vi "Append VI List of SubVIs to Report (refnum).vi"(0 "report in":refnum<class "NI_report.lvclass">, 2 "image format (jpeg)":enum32{"PNG", "JPEG", "GIF"}(ring)=enum."JPEG", 5 "VI":refnum<vi>, 7 "alignment (default)":T2, 9 "include Express VI configuration information (F)":bool, 11 "error in (no error)":errorcluster, 12 "MS Office parameters":T1) -> (4 "report out":refnum<class "NI_report.lvclass">, 6 "VI out":refnum<vi>, 8 "start out (Word)":i32, 10 "end out (Word)":i32, 15 "error out":errorcluster)   [LabVIEW 2020, in "NI_ReportGenerationCore.lvlib"]
doc: "Appends a list of subVIs of the VI you specify in <B>VI</B> to a report. The list includes subVI icons, names, and paths. Wire data to the <B>VI</B> input to determine the polymorphic instance to use or manually select the instance."
uses:
  <vilib>/Utility/NIReport.llb/NI_ReportGenerationCore.lvlib
  <vilib>/Utility/NIReport.llb/NI_report.lvclass
  <vilib>/Utility/NIReport.llb/HTML Report Image Alignment.ctl
  <vilib>/printing/ReportDocExtensions.llb/File_types_for_reports.ctl
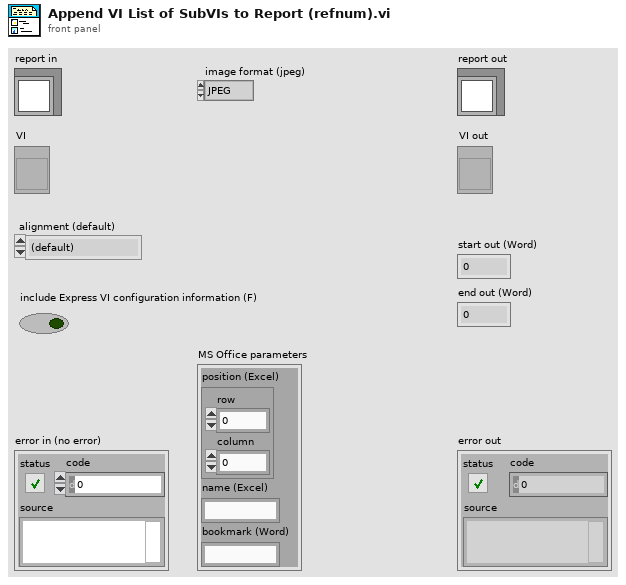
[diagram p1: front panel]
types:
  T1 = cluster{"position (Excel)":cluster{"row":i32, "column":i32}, "name (Excel)":string, "bookmark (Word)":string}
  T2 = typedef "NI_ReportGenerationCore.lvlib/HTML Report Image Alignment.ctl" = enum16{"(default)", "LEFT", "RIGHT", "TOP", "TEXTTOP", "MIDDLE", "ABSMIDDLE", "BASELINE", "BOTTOM", "ABSBOTTOM"}
  T3 = enum8{"No dynamic dispatch VIs", "Include nearest implementation", "Include all overrides"}
  T4 = typedef "NI_ReportGenerationCore.lvlib/File_types_for_reports.ctl" = enum16{".jpg", ".png", ".html", ".gif"}
  T5 = enum32{"invalid app kind", "Development System", "Run Time System", "Student Edition", "Embedded LabVIEW", "Evaluation", "Custom"}
  T6 = enum32{"invalid VI type", "Standard VI", "Control VI", "Global VI", "Polymorphic VI", "Configuration VI", "SubSystem", "Facade VI", "Method VI", "Statechart Diagram VI"}
  T7 = enum16{"Standard Report", "HTML", "Word", "Excel"}
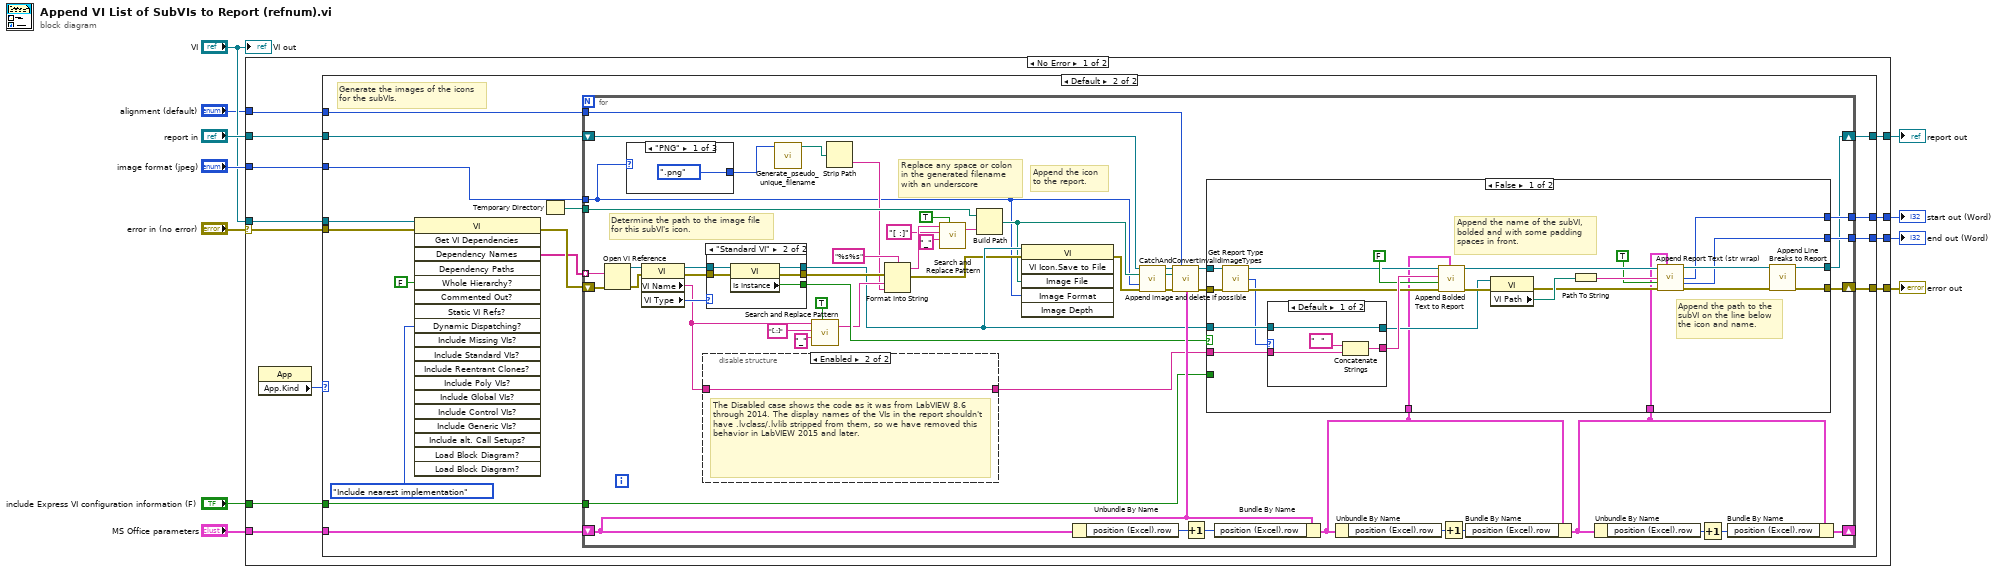
[diagram p0: block diagram]
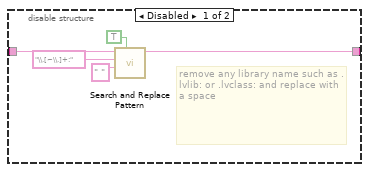
[diagram p3: hidden frame]
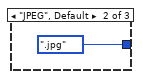
[diagram p4: hidden frame]
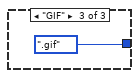
[diagram p5: hidden frame]
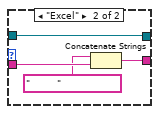
[diagram p6: hidden frame]
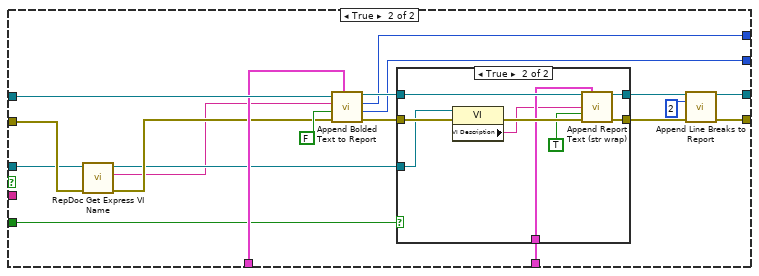
[diagram p7: hidden frame]
diagram:
  n1 = case shown="No Error" "error in (no error)" {
    selector: "error in (no error)" -> [w21 w173]
    tunnel: [w23 w173] -> w10
    tunnel: [w13 w172] -> w8
    tunnel: "report in" -> [w14 w172]
    tunnel: "VI" -> [w22 _]
    tunnel: "image format (jpeg)" -> [w20 _]
    tunnel: "alignment (default)" -> [w19 _]
    tunnel: "MS Office parameters" -> [w18 _]
    tunnel: [w17 _] -> w3
    tunnel: [w16 _] -> w2
    tunnel: "include Express VI configuration information (F)" -> [w15 _]
    frame No Error {
      n2 = property class="App"() -> ("App.Kind"=w12:T5)  [unwired: 2 in, 2 out]
      n3 = case shown="Default" w12 {
        tunnel: [w25 w41] -> w23
        tunnel: w22 -> [_ w39]
        tunnel: w21 -> [w25 w29]
        tunnel: w20 -> [_ w38]
        tunnel: w19 -> [_ w37]
        tunnel: w18 -> [_ w36]
        tunnel: [_ w35] -> w17
        tunnel: [_ w34] -> w16
        tunnel: w15 -> [_ w33]
        tunnel: w14 -> [w24 w32]
        tunnel: [w24 w31] -> w13
        frame "Run Time System" {
          # "Do not try to append\nif running in an\nexecutable"
        }
        frame Default {
          # "Generate the images of the icons\nfor the subVIs."
          n4 = invoke class="VI" method="Get VI Dependencies"(reference=w39, error in=w29, "Whole Hierarchy?"=FALSE, "Dynamic Dispatching?"=T3."Include nearest implementation") -> (error out=w40:errorcluster, "Dependency Names"=w28:string[])  [unwired: 15 in, 17 out]
          n5 = Temporary Directory() -> (w30:path)
          n6 = for {
            shift-right: [w93] -> w41
            shift-left: w40 -> [w91]
            tunnel: w28 -> [w92] mode=indexing
            tunnel: w30 -> [w89]
            tunnel: w38 -> [w43]
            tunnel: w37 -> [w84]
            tunnel: [w83] -> w35
            tunnel: [w82] -> w34
            shift-right: [w71] -> _
            shift-left: w36 -> [w79]
            tunnel: w33 -> [w65]
            shift-right: [w64] -> w31
            shift-left: w32 -> [w63]
            # "Replace any space or colon\nin the generated filename\nwith an underscore"
            # "Append the icon\nto the report."
            # "Determine the path to the image file\nfor this subVI's icon."
            n7 = Open VI Reference(vi path=w92, error in (no error)=w91) -> (vi reference=w90:refnum<vi>, error out=w88:errorcluster)  [unwired: 4 out]
            n8 = case shown="\"PNG\"" w43 {
              tunnel: [File_types_for_reports.".png" ("file type(.jpg)") File_types_for_reports.".jpg" ("file type(.jpg)") File_types_for_reports.".gif" ("file type(.jpg)")] -> w42
              frame "PNG" {
              }
              frame "JPEG", Default {
              }
              frame "GIF" {
              }
            }
            n9 = property class="VI"(reference=w90, error in=w88) -> (reference out=w68:refnum<vi>, error out=w69:errorcluster, "VI Name"=w46:string, "VI Type"=w62:T6)
            n10 = disable-structure shown="Enabled" {
              disable-tunnel: [w98 w99] -> w61
              disable-tunnel: w46 -> [w94 w99]
              frame Disabled {
                # "remove any library name such as .lvlib: or .lvclass: and replace with a space"
                n11 = call <vilib>:"Search and Replace Pattern.vi"("string"=w94, "regular expression (\"\")"="\\.[~\\.]+:" ("regular expression (\"\")"), "replace string (\"\")"=" " ("replace string (\"\")"), "replace all? (F)"=TRUE) -> ("result string"=w98:string)  [unwired: 2 out]
              }
              frame Enabled {
                # "The Disabled case shows the code as it was from LabVIEW 8.6 through 2014. The display names of the VIs in the report shouldn't have .lvclass/.lvlib stripped from them, so we have removed this behavior in LabVIEW 2015 and later."
              }
            }
            n12 = case shown="\"Standard VI\"" w62 {
              tunnel: w69 -> [w166 w171]
              tunnel: w68 -> [w165 w170]
              tunnel: [w166 w169] -> w67
              tunnel: [_ w168] -> w66
              tunnel: [w165 w167] -> w50
              frame Default {
              }
              frame "Standard VI" {
                n13 = property class="VI"(reference=w170, error in=w171) -> (reference out=w167:refnum<vi>, error out=w169:errorcluster, "Is Instance"=w168:bool)
              }
            }
            n14 = call <vilib>:"Generate_pseudo_unique_filename.vi"("file type(.jpg)"=w42) -> ("generated path"=w45:path)  [unwired: 8 in, 2 out]
            n15 = call <vilib>:"Search and Replace Pattern.vi"("string"=w46, "regular expression (\"\")"="[.:]" ("regular expression (\"\")"), "replace string (\"\")"="_" ("replace string (\"\")"), "replace all? (F)"=TRUE) -> ("result string"=w51:string)  [unwired: 2 out]
            n16 = Strip Path(path=w45) -> (name=w44:string)  [unwired: 1 out]
            n17 = Format Into String(format string="%s%s", error in=w67, w51, w44) -> (resulting string=w58:string, error out=w49:errorcluster)  [unwired: 1 in]
            n18 = call <vilib>:"Search and Replace Pattern.vi"("string"=w58, "regular expression (\"\")"="[ :]" ("regular expression (\"\")"), "replace string (\"\")"="_" ("replace string (\"\")"), "replace all? (F)"=TRUE) -> ("result string"=w60:string)  [unwired: 2 out]
            n19 = Build Path(base path=w89, name or relative path=w60) -> (appended path=w47:path)
            n20 = invoke class="VI" method="VI Icon.Save to File"(reference=w50, error in=w49, "Image File"=w47, "Image Format"=w43) -> (error out=w48:errorcluster)  [unwired: 2 in, 5 out]
            n21 = Unbundle By Name(w79) -> ("position (Excel).row"=w81:i32)
            n22 = call-dynamic "CatchAndConvertInvalidImageTypes.vi"("report in"=w63, "path to image"=w47, "image format (jpeg)"=w43, "error in (no error)"=w48) -> ("report out"=w86:refnum<class "NI_report.lvclass">, "path to image out"=w87:path, "error out"=w85:errorcluster)  [unwired: 9 out]
            n23 = call-dynamic "Append image and delete if possible.vi"("report in"=w86, "alignment (default)"=w84, "path to image"=w87, "error in (no error)"=w85, "MS Office parameters"=w79) -> ("report out"=w77:refnum<class "NI_report.lvclass">, "error out"=w78:errorcluster)  [unwired: 1 in, 8 out]
            n24 = Increment(x=w81) -> (x+1=w80:i32)
            n25 = Bundle By Name(cluster=w79, "position (Excel).row"=w80) -> (w74:T1)
            n26 = Unbundle By Name(w74) -> ("position (Excel).row"=w75:i32)
            n27 = Increment(x=w75) -> (x+1=w76:i32)
            n28 = Bundle By Name(cluster=w74, "position (Excel).row"=w76) -> (w70:T1)
            n29 = case shown="False" w66 {
              tunnel: [w126 w146] -> w93
              tunnel: [w110 w143] -> w83
              tunnel: [w109 w142] -> w82
              tunnel: w78 -> [w121 w140]
              tunnel: w77 -> [w120 w153]
              tunnel: w74 -> [w116 w152]
              tunnel: w70 -> [w104 w141]
              tunnel: w61 -> [w115 _]
              tunnel: w50 -> [w114 w138]
              tunnel: w65 -> [_ w150]
              tunnel: [w103 w135] -> w64
              frame False {
                # "Append the path to the\nsubVI on the line below\nthe icon and name."
                # "Append the name of the subVI,\nbolded and with some padding\nspaces in front."
                n30 = call-dynamic "Get Report Type.vi"("report in"=w120, "error in (no error)"=w121) -> ("report out"=w119:refnum<class "NI_report.lvclass">, "report type"=w113:T7, "error out"=w118:errorcluster)  [unwired: 11 out]
                n31 = case shown="Default" w113 {
                  tunnel: w115 -> [w128 w134]
                  tunnel: [w127 w132] -> w124
                  tunnel: w114 -> [w130 w131]
                  tunnel: [w130 w131] -> w117
                  frame Default {
                    n32 = Concatenate Strings("  ", w128) -> (w127:string)
                  }
                  frame "Excel" {
                    n33 = Concatenate Strings("         ", w134) -> (w132:string)
                  }
                }
                n34 = call <vilib>:"Append Bolded Text to Report.vi"("MS Office parameters"=w116, "error in"=w118, "On new line?"=FALSE ("append on new line? (F)"), "Text"=w124, "report in"=w119) -> ("error out"=w122:errorcluster, "report out"=w112:refnum<class "NI_report.lvclass">)  [unwired: 2 out]
                n35 = property class="VI"(reference=w117, error in=w122) -> (error out=w107:errorcluster, "VI Path"=w125:path)  [unwired: 1 out]
                n36 = Path To String(path=w125) -> (string=w106:string)
                n37 = call <vilib>:"Append Report Text (str wrap).vi"("report in"=w112, "MS Office parameters"=w104, "text"=w106, "append on new line? (F)"=TRUE, "error in (no error)"=w107) -> ("report out"=w111:refnum<class "NI_report.lvclass">, "start out (Word)"=w110:i32, "end out (Word)"=w109:i32, "error out"=w108:errorcluster)  [unwired: 1 in, 6 out]
                n38 = call <vilib>:"Append Line Breaks to Report.vi"("report in"=w111, "error in (no error)"=w108) -> ("report out"=w103:refnum<class "NI_report.lvclass">, "error out"=w126:errorcluster)  [unwired: 1 in, 11 out]
              }
              frame True {
                n39 = call <vilib>:"RepDoc Get Express VI Name.vi"("error in (no error)"=w140, "VI Refnum"=w138) -> ("error out"=w139:errorcluster, "Express VI Name"=w136:string, "dup VI Refnum"=w137:refnum<vi>)  [unwired: 7 out]
                n40 = call <vilib>:"Append Bolded Text to Report.vi"("MS Office parameters"=w152, "error in"=w139, "On new line?"=FALSE, "Text"=w136, "report in"=w153) -> ("error out"=w149:errorcluster, "end out (Word)"=w142:i32, "start out (Word)"=w143:i32, "report out"=w148:refnum<class "NI_report.lvclass">)
                n41 = case shown="True" w150 {
                  tunnel: w149 -> [w155 w164]
                  tunnel: w148 -> [w154 w159]
                  tunnel: [w155 w162] -> w147
                  tunnel: [w154 w160] -> w145
                  tunnel: w141 -> [_ w158]
                  tunnel: w137 -> [_ w163]
                  frame False {
                    # "Do not include Express\nVI Config Information."
                  }
                  frame True {
                    n42 = property class="VI"(reference=w163, error in=w164) -> (error out=w161:errorcluster, "VI Description"=w157:string)  [unwired: 1 out]
                    n43 = call <vilib>:"Append Report Text (str wrap).vi"("report in"=w159, "MS Office parameters"=w158, "text"=w157, "append on new line? (F)"=TRUE, "error in (no error)"=w161) -> ("report out"=w160:refnum<class "NI_report.lvclass">, "error out"=w162:errorcluster)  [unwired: 1 in, 8 out]
                  }
                }
                n44 = call <vilib>:"Append Line Breaks to Report.vi"("report in"=w145, "number of line breaks"=u32 2 ("Number of line breaks"), "error in (no error)"=w147) -> ("report out"=w135:refnum<class "NI_report.lvclass">, "error out"=w146:errorcluster)  [unwired: 11 out]
              }
            }
            n45 = Unbundle By Name(w70) -> ("position (Excel).row"=w73:i32)
            n46 = Increment(x=w73) -> (x+1=w72:i32)
            n47 = Bundle By Name(cluster=w70, "position (Excel).row"=w72) -> (w71:T1)
          }
        }
      }
    }
    frame Error {
    }
  }
  "error out" <- w10
  "report out" <- w8
  "start out (Word)" <- w3
  "end out (Word)" <- w2
  "VI out" <- "VI"
